vi "XYZ Stage - Setup.vi"(8 "error in (no error)":errorcluster) -> (0 "error out":errorcluster, 2 "Stage Comms":T1={"CommsProtocol.lvclass"=refnum, "CommsProtocol.lvclass 2"=refnum, "CommsProtocol.lvclass 3"=refnum, "XYZ Control Config"=enum."XYZ", "Translation Stage Description"=""}, 3 "XYZ Stage Control.lvclass":refnum<class "XYZ Stage Control.lvclass">)   [LabVIEW 2020]
uses:
  typedefs/TranslationStageControlInfo.ctl
  Generic Comms/CommsProtocol/CommsProtocol.lvclass
  typedefs/XYZControlConfig.ctl
  XYZ Stage Control/XYZ Stage Control.lvclass
  Typedefs/HW config states enum.ctl
  Scientifica XYZ Gen1/Scientifica XYZ Gen1.lvclass
  Serial Comms/Serial Comms/Serial Comms.lvclass
  C:/LV_unversioned_SP/local_copy_ml_yale/Peripherals Control/Generic Comms/CommsProtocol/CommsProtocol.lvclass
  Serial Comms/Serial - Settings.ctl
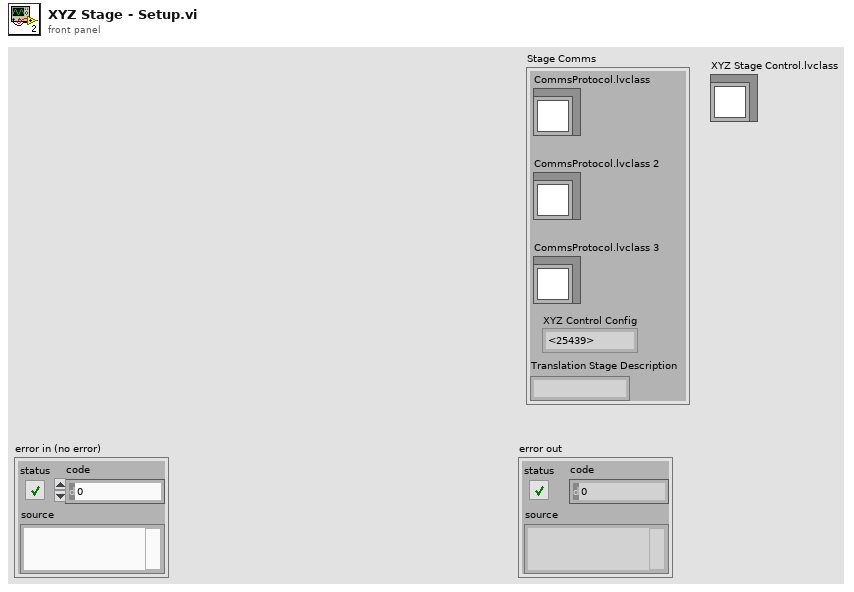
[diagram p1: front panel]
types:
  T1 = typedef "TranslationStageControlInfo.ctl" = cluster{"CommsProtocol.lvclass":refnum<class "CommsProtocol.lvclass">, "CommsProtocol.lvclass 2":refnum<class "CommsProtocol.lvclass">, "CommsProtocol.lvclass 3":refnum<class "CommsProtocol.lvclass">, "XYZ Control Config":T2, "Translation Stage Description":string}
  T2 = typedef "XYZControlConfig.ctl" = enum16{"None", "XYZ", "XY-Z", "X-Y-Z", "Z"}
  T3 = typedef "HW config states enum.ctl" = enum16{"Load from file", "Save to file", "Write all", "Read all", "Write XY stage settings", "Write DAQ FPGA settings", "Write Control FPGA settings", "Write Phys Channels", "Write System Config", "Write HW Config", "Save System Config", "Save HW Config", "Clear", "Compare from file"}
  T4 = typedef "Hardware Configuration settings.ctl" = cluster{"Dev. PC":bool, "Swap XY on stage":bool, "No of AOD":u8, "MC Supported":bool, "Axial MC":bool, "Computer MAC address":string, "Externalise Triggers":bool, "Trigger HW config":T5, "DAQmx Chan":T6, "XYZ Stage Control Config":T2, "XY stage available":bool, "XY Comms Config Cluster":T7, "Y stage available":bool, "Y Comms Config Cluster":T7, "Z stage available":bool, "Z Comms Config Cluster ":T7, "Encoder available":bool, "Encoder":T9, "VidRec available":bool, "Cam VidRec":T10, "Laser Power Control HW config":T11, "Laser 1 available":bool, "Laser 1 config cluster":T12, "Prechirper 1 available":bool, "Prechirper 1 config cluster":T13, "Control system.FPGA available?":bool, "Control Sys. HW config":T14, "DAQ FPGA HW Config":T15, "PMT Control Voltage Limits":T19}
  T5 = typedef "Triggers HW config.ctl" = cluster{"Available Device List":i32, "Device Address":string}
  T6 = typedef "DAQmx physical channels cluster.ctl" = cluster{"Pockels AO":tag, "Hard shutter AO":tag, "PMT AOs":tag, "Galvo AOs":tag, "Power meter AI":tag}
  T7 = typedef "Peripherals comms config cluster.ctl" = cluster{"Name":string, "Device Address":string, "Port ":u16, "Baudrate":i32, "Comms Type":T8}
  T8 = typedef "Comms Type.ctl" = enum16{"GPIB-IEEE488", "Serial-RS232", "Serial-RS485", "Serial-RS422", "Serial-USB", "Ethernet-TCP/IP", "Ethernet-UDP"}
  T9 = typedef "Encoder config cluster.ctl" = cluster{"IP address":string, "Port":u16, "Wheel radius (cm)":dbl, "Encoder Trigger":tag}
  T10 = typedef "Cam VidRec HW config setup cluster.ctl" = cluster{"DO flag-Video record":tag, "DO flag-Trial start":tag}
  T11 = typedef "Laser Power Control HW config.ctl" = cluster{"Laser Power Control":string, "Laser Power Modulation Control":enum16{"NI", "FPGA"}}
  T12 = typedef "Laser 1 config cluster.ctl" = cluster{"COM port":refnum<visa-resource-name>, "Baud Rate":i32, "Type":string}
  T13 = typedef "PreChirper 1 config cluster.ctl" = cluster{"Type":string, "Baud Rate":i32, "COM port":refnum<visa-resource-name>}
  T14 = typedef "Control Sys HW config cluster.ctl" = cluster{"Control system.FPGA Type":enum16{"Virtex 5", "Virtex 7"}, "Control system.Network adapter name":string, "Control system.MAC address":string, "Control system.Ethernet Port":u32, "Control system.Ethernet Port Opened":bool}
  T15 = typedef "DAQ FPGA HW config cluster.ctl" = cluster{"FGPA Ref":T16, "Target":T17, "input card type":T18}
  T16 = typedef "FPGA Ref.ctl" = refnum<k20>
  T17 = typedef "nirio_resource_hc.ctl" = tag
  T18 = typedef "FPGA input type AC-DC.ctl" = enum16{"AC Card", "DC Card"}
  T19 = typedef "PMT Control Voltage limits.ctl" = cluster{"Lower Limit":dbl, "Upper Limit":dbl}
  T20 = typedef "Serial - Settings.ctl" = cluster{"VISA resource name ":refnum<visa-resource-name>, "baud rate":u32, "data bits":u16, "parity":enum16{"None", "Odd", "Even", "Mark", "Space"}, "stop bits":u16, "flow control":u16, "Timeout":u32, "termination char\n(0xA = '\\n' = LF) ":u8, "Enable Termination Character":bool}
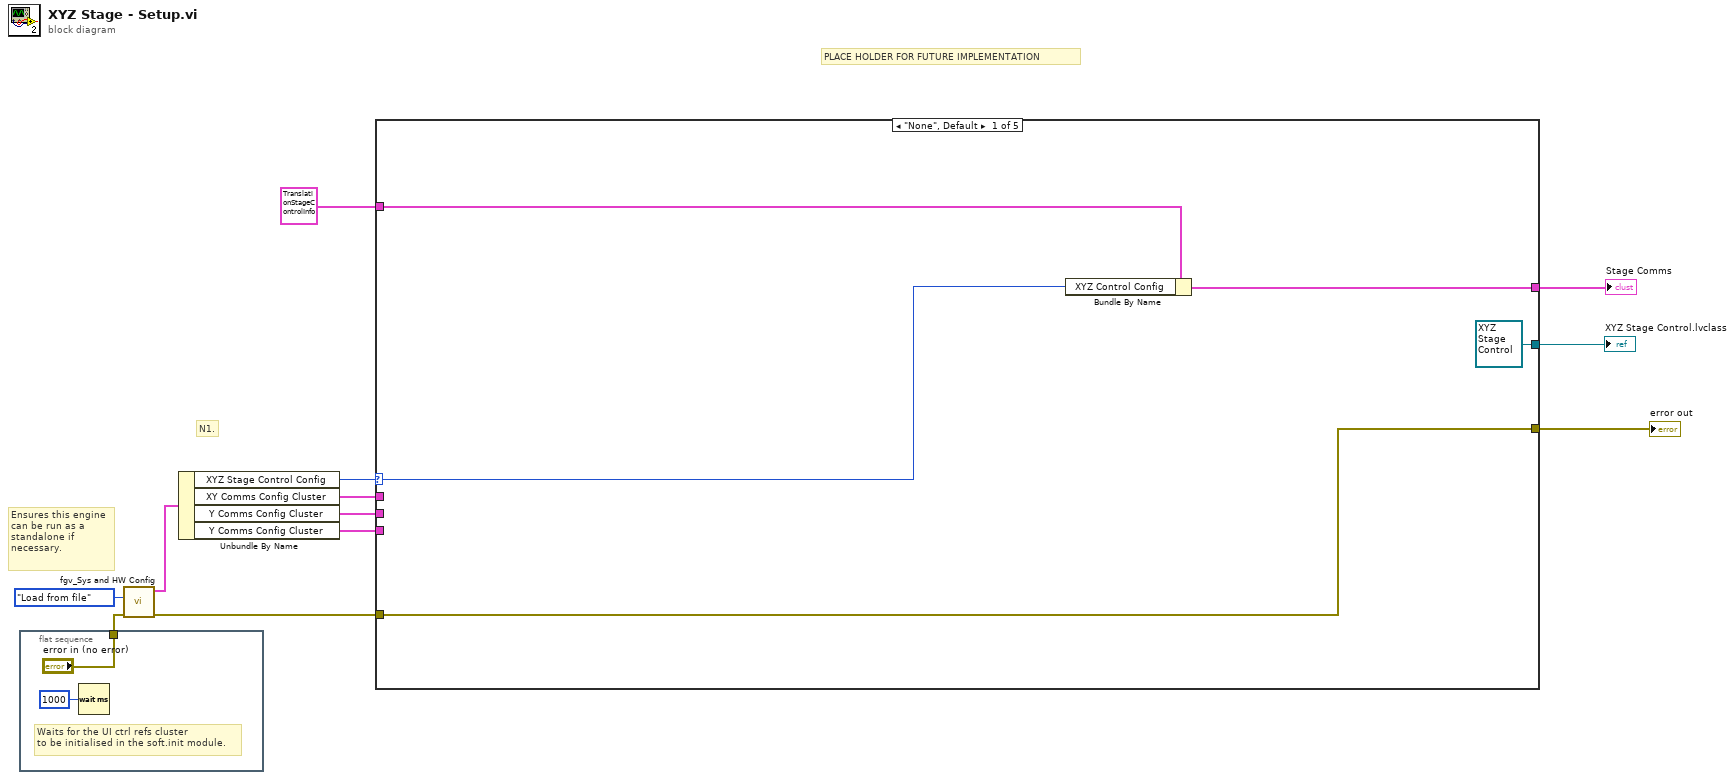
[diagram p0: block diagram]
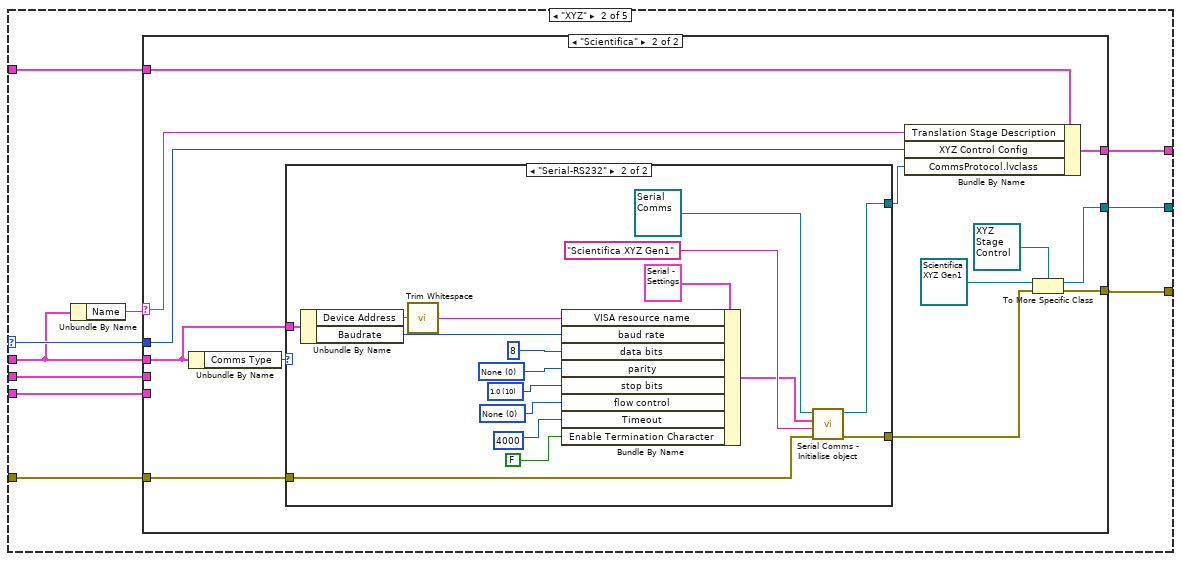
[diagram p2: hidden frame]
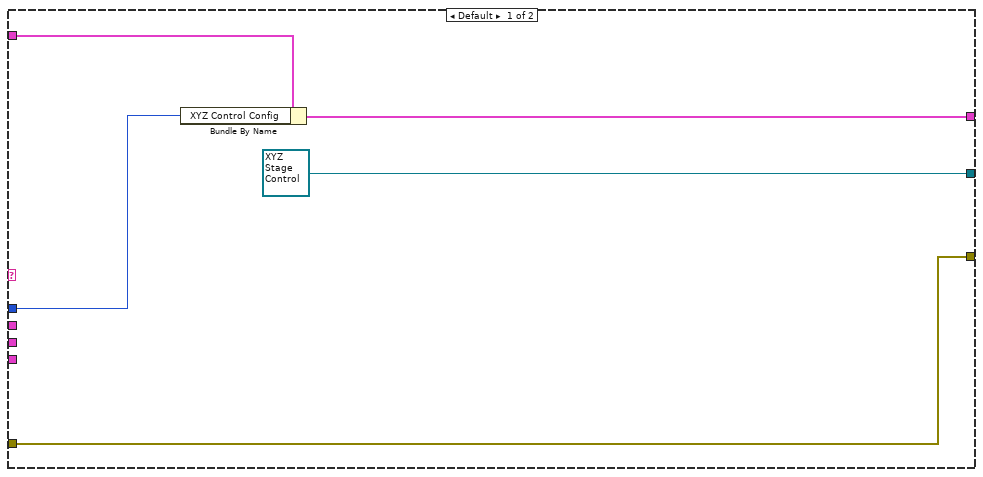
[diagram p3: hidden frame]
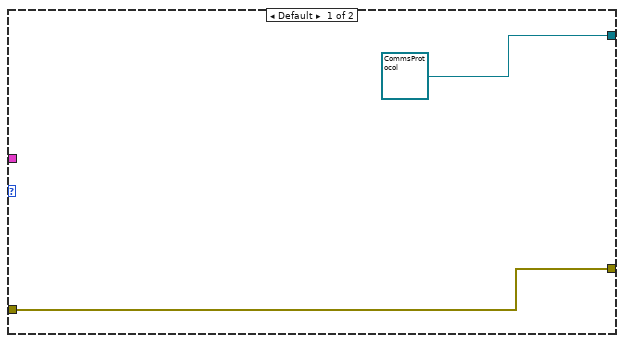
[diagram p4: hidden frame]
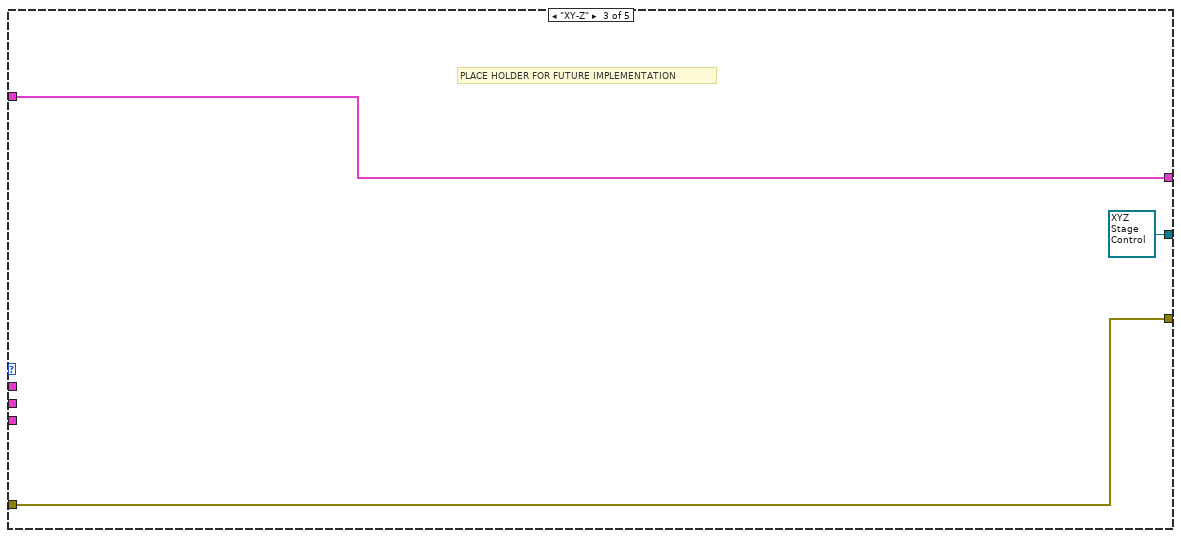
[diagram p5: hidden frame]
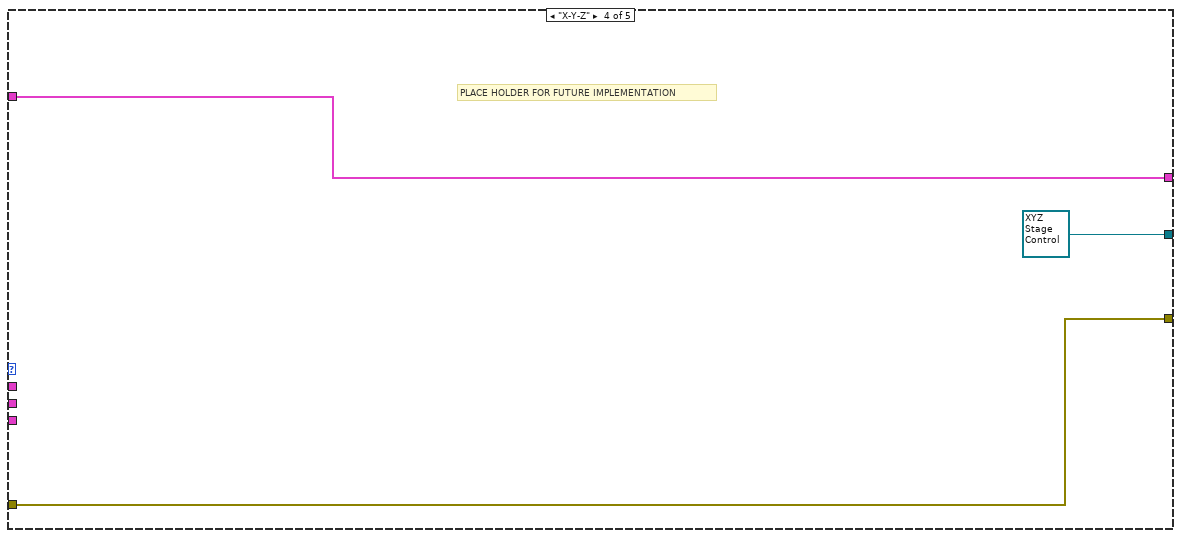
[diagram p6: hidden frame]
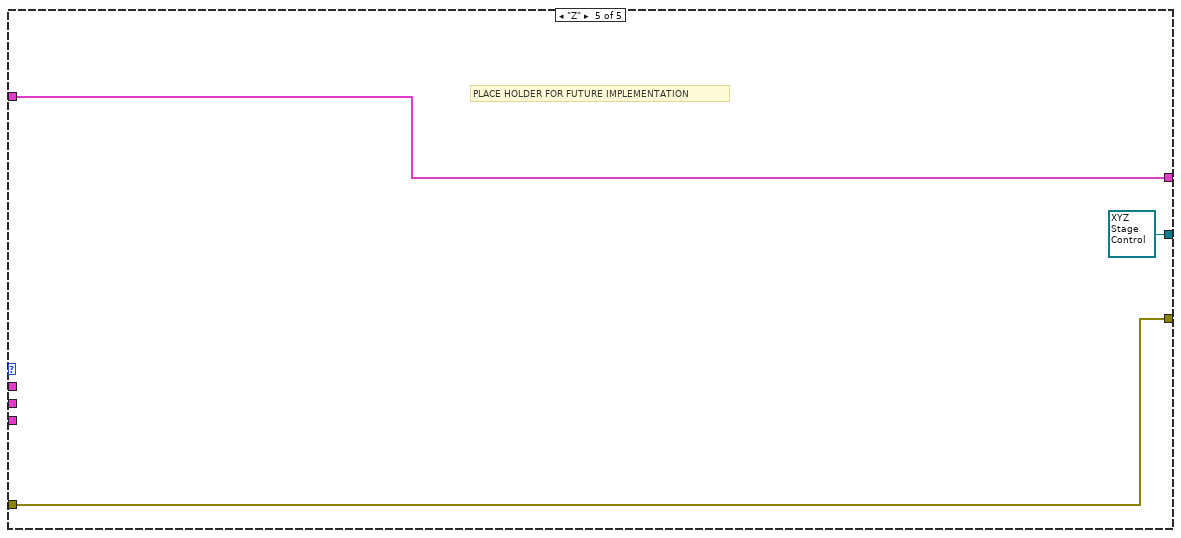
[diagram p7: hidden frame]
diagram:
  # "PLACE HOLDER FOR FUTURE IMPLEMENTATION"
  # "N1."
  # "Ensures this engine can be run as a standalone if necessary."
  n1 = flat-sequence {
    tunnel: ["error in (no error)"] -> w10
    frame #0 {
      # "Waits for the UI ctrl refs cluster\nto be initialised in the soft.init module."
      n2 = Wait (ms)(milliseconds to wait=u32 1000) -> ()  [unwired: 1 out]
    }
  }
  n3 = call "fgv_Sys and HW Config.vi"("Function"=HW_config_states_enum."Load from file", "error in (no error)"=w10) -> ("error out"=w1:errorcluster, "Hardware Configuration OUT"=w11:T4)  [unwired: 7 in, 1 out]
  n4 = Unbundle By Name(w11) -> ("XYZ Stage Control Config"=w6:T2, "XY Comms Config Cluster"=w8:T7, "Y Comms Config Cluster"=w7:T7, "Y Comms Config Cluster"=w4:T7)
  n5 = case shown="\"None\", Default" w6 {
    selector: w6 -> [w15 w25 _ _ _]
    tunnel: [w18 w29 w68 w70 w73] -> w9
    tunnel: w8 -> [_ w22 _ _ _]
    tunnel: w7 -> [_ w28 _ _ _]
    tunnel: T1 {"CommsProtocol.lvclass"=refnum, "CommsProtocol.lvclass 2"=refnum, "CommsProtocol.lvclass 3"=refnum, "XYZ Control Config"=enum."None", "Translation Stage Description"=""} ("Stage Comms") -> [w17 w27 w69 w72 w75]
    tunnel: w4 -> [_ w26 _ _ _]
    tunnel: [w16 w24 w69 w72 w75] -> w3
    tunnel: [refnum<class "XYZ Stage Control.lvclass"> refnum ("XYZ Stage Control.lvclass") w23 refnum<class "XYZ Stage Control.lvclass"> refnum ("XYZ Stage Control.lvclass") refnum<class "XYZ Stage Control.lvclass"> refnum ("XYZ Stage Control.lvclass") refnum<class "XYZ Stage Control.lvclass"> refnum ("XYZ Stage Control.lvclass")] -> w2
    tunnel: w1 -> [w18 w20 w68 w70 w73]
    frame "None", Default {
      n6 = Bundle By Name(cluster=w17, "XYZ Control Config"=w15) -> (w16:T1)
    }
    frame "XYZ" {
      n7 = Unbundle By Name(w22) -> ("Name"=w21:string)
      n8 = case shown="\"Scientifica\"" w21 {
        selector: w21 -> [_ w36]
        tunnel: [w30 w46] -> w29
        tunnel: w22 -> [_ w42]
        tunnel: w28 -> [_ _]
        tunnel: w27 -> [w34 w39]
        tunnel: w26 -> [_ _]
        tunnel: w25 -> [w33 w35]
        tunnel: [w32 w37] -> w24
        tunnel: [refnum<class "XYZ Stage Control.lvclass"> refnum ("XYZ Stage Control.lvclass") w44] -> w23
        tunnel: w20 -> [w30 w41]
        frame Default {
          n9 = Bundle By Name(cluster=w34, "XYZ Control Config"=w33) -> (w32:T1)
        }
        frame "Scientifica" {
          n10 = Unbundle By Name(w42) -> ("Comms Type"=w43:T8)
          n11 = case shown="\"Serial-RS232\"" w43 {
            tunnel: w42 -> [_ w63]
            tunnel: [refnum<class "CommsProtocol.lvclass"> refnum ("CommsProtocol.lvclass") w52] -> w38
            tunnel: w41 -> [w48 w51]
            tunnel: [w48 w50] -> w40
            frame Default {
            }
            frame "Serial-RS232" {
              w56 = u16 0 items=["None"=0, "XON/XOFF"=1, "RTS/CTS"=2, "DTR/DSR"=4] ("flow control")
              w57 = u16 10 items=["1.0"=10, "1.5"=15, "2.0"=20] ("stop bits")
              w58 = u16 0 items=["None", "Odd", "Even", "Mark", "Space"] ("parity")
              n12 = Unbundle By Name(w63) -> ("Device Address"=w62:string, "Baudrate"=w60:i32)
              n13 = call <vilib>:"Trim Whitespace.vi"("string"=w62) -> ("trimmed string"=w61:string)  [unwired: 1 in]
              n14 = Bundle By Name(cluster=T20 {"VISA resource name "="", "baud rate"=9600, "data bits"=8, "parity"=enum."None", "stop bits"=10, "flow control"=0, "Timeout"=0, "termination char\n(0xA = '\\n' = LF) "=10, "Enable Termination Character"=FALSE} ("Serial Settings"), "VISA resource name"=w61, "baud rate"=w60, "data bits"=u16 8, "parity"=w58, "stop bits"=w57, "flow control"=w56, "Timeout"=u32 4000, "Enable Termination Character"=FALSE) -> (w64:T20)
              n15 = call "Serial Comms - Initialise object.vi"("error in (no error)"=w51, "Connection Name"="Scientifica XYZ Gen1", "Serial Settings"=w64, "Serial Comms in"=refnum<class "Serial Comms.lvclass"> refnum ("Serial Comms.lvclass")) -> ("error out"=w50:errorcluster, "Serial Comms out"=w52:refnum<class "Serial Comms.lvclass">)  [unwired: 6 in]
            }
          }
          n16 = Bundle By Name(cluster=w39, "Translation Stage Description"=w36, "XYZ Control Config"=w35, "CommsProtocol.lvclass"=w38) -> (w37:T1)
          n17 = To More Specific Class(target class=refnum<class "XYZ Stage Control.lvclass"> refnum ("XYZ Stage Control.lvclass"), reference=refnum<class "Scientifica XYZ Gen1.lvclass"> refnum ("Scientifica XYZ Gen1.lvclass"), error in=w40) -> (specific class reference=w44:refnum<class "XYZ Stage Control.lvclass">, error out=w46:errorcluster)
        }
      }
    }
    frame "XY-Z" {
      # "PLACE HOLDER FOR FUTURE IMPLEMENTATION"
    }
    frame "X-Y-Z" {
      # "PLACE HOLDER FOR FUTURE IMPLEMENTATION"
    }
    frame "Z" {
      # "PLACE HOLDER FOR FUTURE IMPLEMENTATION"
    }
  }
  "Stage Comms" <- w3
  "XYZ Stage Control.lvclass" <- w2
  "error out" <- w9
